vi "Point_Read_point.vi"(8 "Error In":errorcluster, 10 "Tag":string, 11 "Map":T3) -> (0 "Error Out":errorcluster, 1 "Point":T1, 2 "Found?":bool, 3 "Map Out":T3)   [LabVIEW 2017, in "PointValueMap.lvlib"]
uses:
  <vilib>/addons/PointValueMap/PointValueMap.lvlib
  <vilib>/addons/PointValueMap/controls/PointMap.ctl
  <vilib>/addons/PointValueMap/controls/Point.ctl
  <vilib>/addons/PointValueMap/controls/DataTypes.ctl
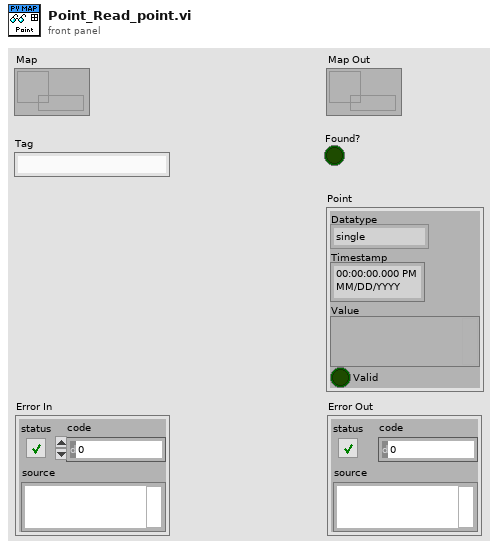
[diagram p1: front panel]
types:
  T1 = typedef "PointValueMap.lvlib/Point.ctl" = cluster{"Datatype":T2, "Timestamp":timestamp, "Value":variant, "Valid":bool}
  T2 = typedef "PointValueMap.lvlib/DataTypes.ctl" = enum16{"single", "double", "i32", "string", "variant"}
  T3 = typedef "PointValueMap.lvlib/PointMap.ctl" = refnum<data-value>
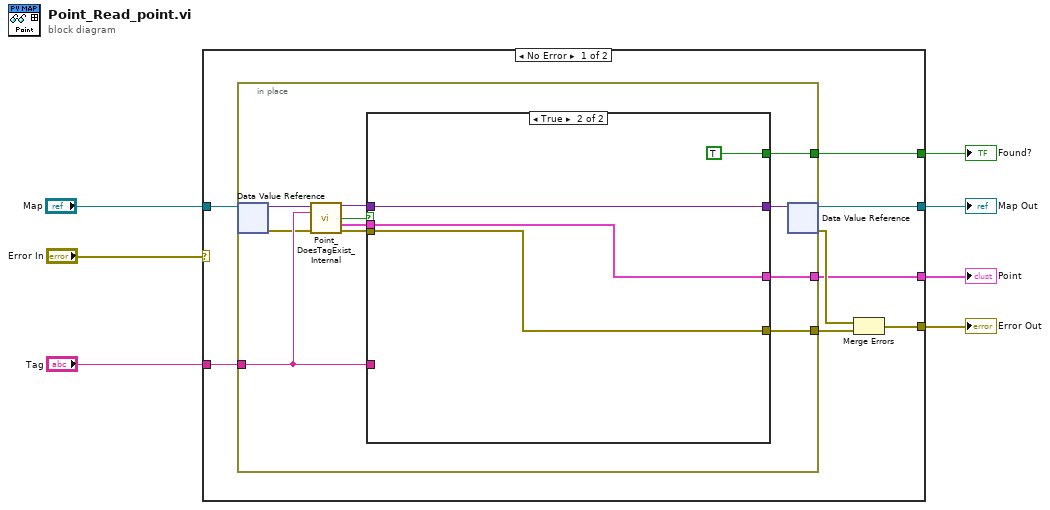
[diagram p0: block diagram]
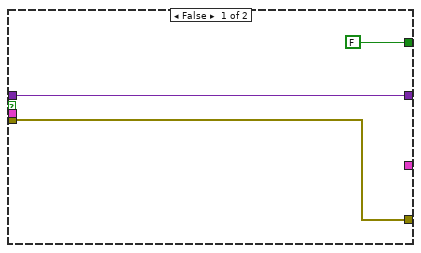
[diagram p2: hidden frame]
diagram:
  n1 = case shown="No Error" "Error In" {
    selector: "Error In" -> [_ w35]
    tunnel: "Map" -> [w15 w34]
    tunnel: "Tag" -> [w14 _]
    tunnel: [w12 w35] -> w6
    tunnel: [w11 w34] -> w3
    tunnel: [w9 _] -> w2
    tunnel: [w8 _] -> w1
    frame No Error {
      n2 = in-place {
        in-place-border: w14 -> [w23]
        in-place-border: [w25] -> w13
        in-place-border: [w17] -> w9
        in-place-border: [w16] -> w8
        n3 = in-place-dvr #1(w15) -> (w24:variant, w19:errorcluster)
        n4 = call <vilib>:"Point_DoesTagExist_Internal.vi"("Map"=w24, "Tag"=w23, "Error In"=w19) -> ("Map Out"=w21:variant, "Tag Exists"=w22:bool, "Point"=w18:T1, "Error Out"=w20:errorcluster)  [unwired: 7 in, 2 out]
        n5 = case shown="True" w22 {
          tunnel: [w29 w33] -> w26
          tunnel: [w28 w32] -> w25
          tunnel: w21 -> [w29 w33]
          tunnel: w20 -> [w28 w32]
          tunnel: w23 -> [_ _]
          tunnel: w18 -> [_ w31]
          tunnel: [_ w31] -> w17
          tunnel: [FALSE TRUE] -> w16
          frame False {
          }
          frame True {
          }
        }
        n6 = in-place-dvr #1(w26) -> (w11:T3, w10:errorcluster)
      }
      n7 = Merge Errors(w10, w13) -> (w12:errorcluster)
    }
    frame Error {
    }
  }
  "Error Out" <- w6
  "Map Out" <- w3
  "Point" <- w2
  "Found?" <- w1
